vi "COTP - Called TSAP Parameter.vi"(10 "Rack No.":u8 format="%0d", 11 "Slot No.":u8 format="%0d") -> (3 "COTP Called TSAP":T1=[194, 2, 3, 0] format="0x%02x")   [LabVIEW 2014, in "S7NetCom.lvclass"]
doc: "ISO DP 8073 (RFC 905) Header bytes constant for \"Connection Request\" PDU type. \n_____\nCopyright (c) 2019 Hampel Software Engineering (HSE), released under BSD license. More info can be found on https://dokuwiki.hampel-soft.com/code/hse/s7netcom. Original code published by Marc Christenson, Sisu Devices."
uses:
  S7NetCom.lvclass
  Controls/S7NetCom_HexByteArray.ctl
  Controls/S7NetCom_HexByte.ctl
panel:
  # "More info on https://dokuwiki.hampel-soft.com/code/hse/s7netcom\n\nCopyright (c) 2019, HAMPEL SOFTWARE ENGINEERING (HSE)\nOriginal code developed by Marc Christenson, Sisu Devices\nAll rights reserved.\n\nRedistribution and use in source and binary forms, with or without\nmodification, are permitted provided that the following conditions are met:\n\n1. Redistributions of source code must retain the above copyright\n   notice, this list of conditions and the following disclaimer.\n\n2. Redistributions in binary form must reproduce the above copyright\n   notice, this list of conditions and the following disclaimer in the\n   documentation and/or other materials provided with the distribution.\n\n3. All advertising materials mentioning features or use of this software\n   must display the following acknowledgement:\n   This product includes software developed by HAMPEL SOFTWARE ENGINEERING.\n\n4. Neither the name of HAMPEL SOFTWARE ENGINEERING nor the\n   names of its contributors may be used to endorse or promote products\n   derived from this software without specific prior written permission.\n\nTHIS SOFTWARE IS PROVIDED BY HAMPEL SOFTWARE ENGINEERING ''AS IS'' AND ANY\nEXPRESS OR IMPLIED WARRANTIES, INCLUDING, BUT NOT LIMITED TO, THE IMPLIED\nWARRANTIES OF MERCHANTABILITY AND FITNESS FOR A PARTICULAR PURPOSE ARE\nDISCLAIMED. IN NO EVENT SHALL HAMPEL SOFTWARE ENGINEERING BE LIABLE FOR ANY\nDIRECT, INDIRECT, INCIDENTAL, SPECIAL, EXEMPLARY, OR CONSEQUENTIAL DAMAGES\n(INCLUDING, BUT NOT LIMITED TO, PROCUREMENT OF SUBSTITUTE GOODS OR SERVICES;\nLOSS OF USE, DATA, OR PROFITS; OR BUSINESS INTERRUPTION) HOWEVER CAUSED AND\nON ANY THEORY OF LIABILITY, WHETHER IN CONTRACT, STRICT LIABILITY, OR TORT\n(INCLUDING NEGLIGENCE OR OTHERWISE) ARISING IN ANY WAY OUT OF THE USE OF THIS\nSOFTWARE, EVEN IF ADVISED OF THE POSSIBILITY OF SUCH DAMAGE."
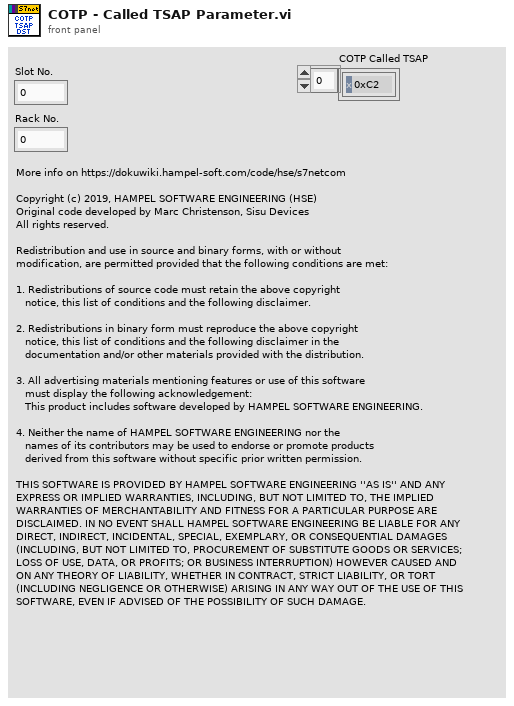
[diagram p1: front panel]
types:
  T1 = typedef "S7NetCom.lvclass/S7NetCom_HexByteArray.ctl" = T2[]
  T2 = typedef "S7NetCom.lvclass/S7NetCom_HexByte.ctl" = u8
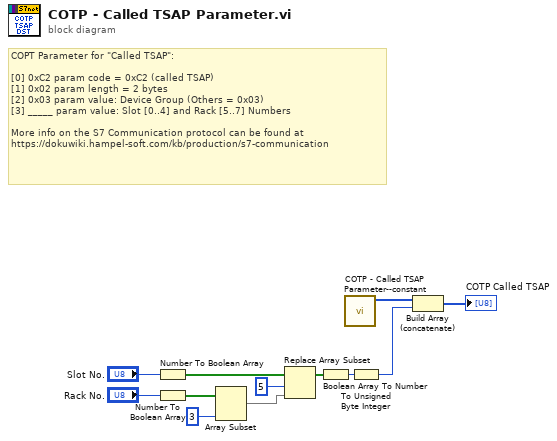
[diagram p0: block diagram]
diagram:
  # "COPT Parameter for \"Called TSAP\":\n\n[0]\t0xC2\tparam code = 0xC2 (called TSAP)\n[1]\t0x02\tparam length = 2 bytes\n[2]\t0x03\tparam value: Device Group (Others = 0x03)\n[3]\t_____\tparam value: Slot [0..4] and Rack [5..7] Numbers\n\nMore info on the S7 Communication protocol can be found at\nhttps://dokuwiki.hampel-soft.com/kb/production/s7-communication"
  n1 = Number To Boolean Array(number="Slot No.") -> (Boolean array=w9:bool[])
  n2 = Number To Boolean Array(number="Rack No.") -> (Boolean array=w5:bool[])
  n3 = Array Subset(array=w5, length=3 ("index")) -> (w4:bool[])  [unwired: 1 in]
  n4 = Replace Array Subset(array=w9, new element=w4, index=5) -> (w8:bool[])
  n5 = Boolean Array To Number(Boolean array=w8) -> (number=w7:u32)
  n6 = call "COTP - Called TSAP Parameter--constant.vi"() -> ("COTP Called TSAP"=w1:T1)  [unwired: 11 in]
  n7 = To Unsigned Byte Integer(number=w7) -> (unsigned 8bit integer=w6:u8)
  n8 = Build Array (concatenate)(w1, w6) -> (→"COTP Called TSAP":T1)
